vi "ImageIndexMap.vi"(9 "Pixel Count":u32, 10 "Scan Mode":enum16{"Raster", "Serpentine"}(ring), 11 "Wave Count in":u64) -> (3 "Wave Count out":u64)   [LabVIEW 2020]
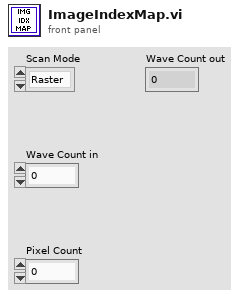
[diagram p1: front panel]
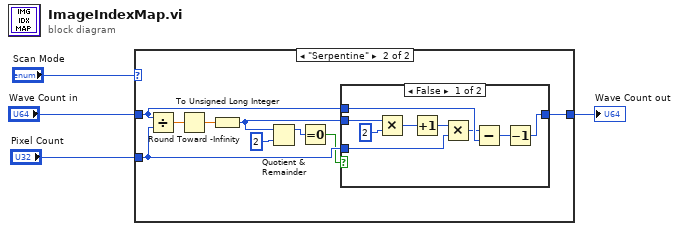
[diagram p0: block diagram]
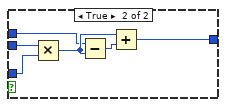
[diagram p3: hidden frame]
diagram:
  n1 = case shown="\"Serpentine\"" "Scan Mode" {
    tunnel: "Wave Count in" -> [w5 w10]
    tunnel: "Pixel Count" -> [_ w9]
    tunnel: [w5 w6] -> w2
    frame "Raster", Default {
    }
    frame "Serpentine" {
      n2 = Divide(x=w10, y=w9) -> (x/y=w12:dbl)
      n3 = Round Toward -Infinity(1:w12) -> (0:w11:dbl)
      n4 = To Unsigned Long Integer(number=w11) -> (unsigned 32bit integer=w7:u32)
      n5 = Quotient & Remainder(x=w7, y=2) -> (x-y*floor(x/y)=w13:u32)  [unwired: 1 out]
      n6 = Equal To 0?(x=w13) -> (x = 0?=w8:bool)
      n7 = case shown="False" w8 {
        tunnel: w7 -> [w23 w29]
        tunnel: w9 -> [w22 w28]
        tunnel: w10 -> [w21 w25]
        tunnel: [w20 w27] -> w6
        frame False {
          n8 = Multiply(x=w23, y=u32 2) -> (x*y=w17:u32)
          n9 = Increment(x=w17) -> (x+1=w16:u32)
          n10 = Multiply(x=w16, y=w22) -> (x*y=w15:u32)
          n11 = Subtract(x=w15, y=w21) -> (x-y=w19:u64)
          n12 = Decrement(x=w19) -> (x-1=w20:u64)
        }
        frame True {
          n13 = Multiply(x=w29, y=w28) -> (x*y=w26:u32)
          n14 = Subtract(x=w25, y=w26) -> (x-y=w24:u64)
          n15 = Add(x=w26, y=w24) -> (x+y=w27:u64)
        }
      }
    }
  }
  "Wave Count out" <- w2
